vi "Main_25a.vi"() -> ()   [LabVIEW 2020]
uses:
  Cluster SNAFU Number.ctl
  ENUM_SNAFU Digit.ctl
  0fccf756-9261-4bff-9dad-ca374a7b94a1.vi
  <vilib>/Comparison/Equal/Equal Functor/Equal Functor.lvclass
panel:
  out "String":string
  in  "Example 2":string="1=-0-2\n12111\n2=0=\n21\n2=01\n111\n20012\n112\n1=-1=\n1-12\n12\n1=\n122"
  out "Array 2":T1[](array[typedef])
  out "Array":i64[](array[numeric])
  in  "Example":string="1=-0-2\n12111\n2=0=\n21\n2=01\n111\n20012\n112\n1=-1=\n1-12\n12\n1=\n122"
  in  "Decimal to SNAFU":string="Decimal          SNAFU\n        1              1\n        2              2\n        3             1=\n        4             1-\n        5             10\n        6             11\n        7             12\n        8             2=\n        9             2-\n       10             20\n       15            1=0\n       20            1-0\n     2022         1=11-2\n    12345        1-0---0\n314159265  1121-1110-1=0"
  out "Answer":i64
  in  "Puzzle":string="11-00\n2--2==212=12\n1=0110121=2\n1=012-21-=121\n1==0-1121-=200=2212\n1=1210===00=\n11210021-0001010-\n12=1-10-1-\n212-2==221-210-21\n1=-01=0-02-2-=-222=\n1=022000===-22010\n1=01=12202\n11=\n202-1\n2-12-2=--1\n10-=-00=101=-0-=-0\n1112-1\n2--1201\n1=1==-020=1-\n1--0-=2-0022-\n1=-1-21-200-102=\n11=100021210\n1=2=01=2-=01-=\n1=0120-11-0-=-2=-2\n1=-20221=2=-2=\n1-0\n1=00=-=11100--=2\n22122\n1=102222\n1210=1=001-=000\n1--200102022-=\n102=12=-1==\n100=\n20-02\n10\n10==-102\n11=020-0210-1-2012=\n12-11=0-1-=\n20=-\n212=1-1-10\n1=20=1-=2-11=0\n1=22\n120=2202=12200\n1-0-1\n211011-11=\n2=120=--==0==--0-0\n110-0-=-10-1-112\n1=2=1-=1-2\n1=12==10\n10=2110..."
  in  "SNAFU to Decimal":string="SNAFU  Decimal\n1=-0-2     1747\n 12111      906\n  2=0=      198\n    21       11\n  2=01      201\n   111       31\n 20012     1257\n   112       32\n 1=-1=      353\n  1-12      107\n    12        7\n    1=        3\n   122       37"
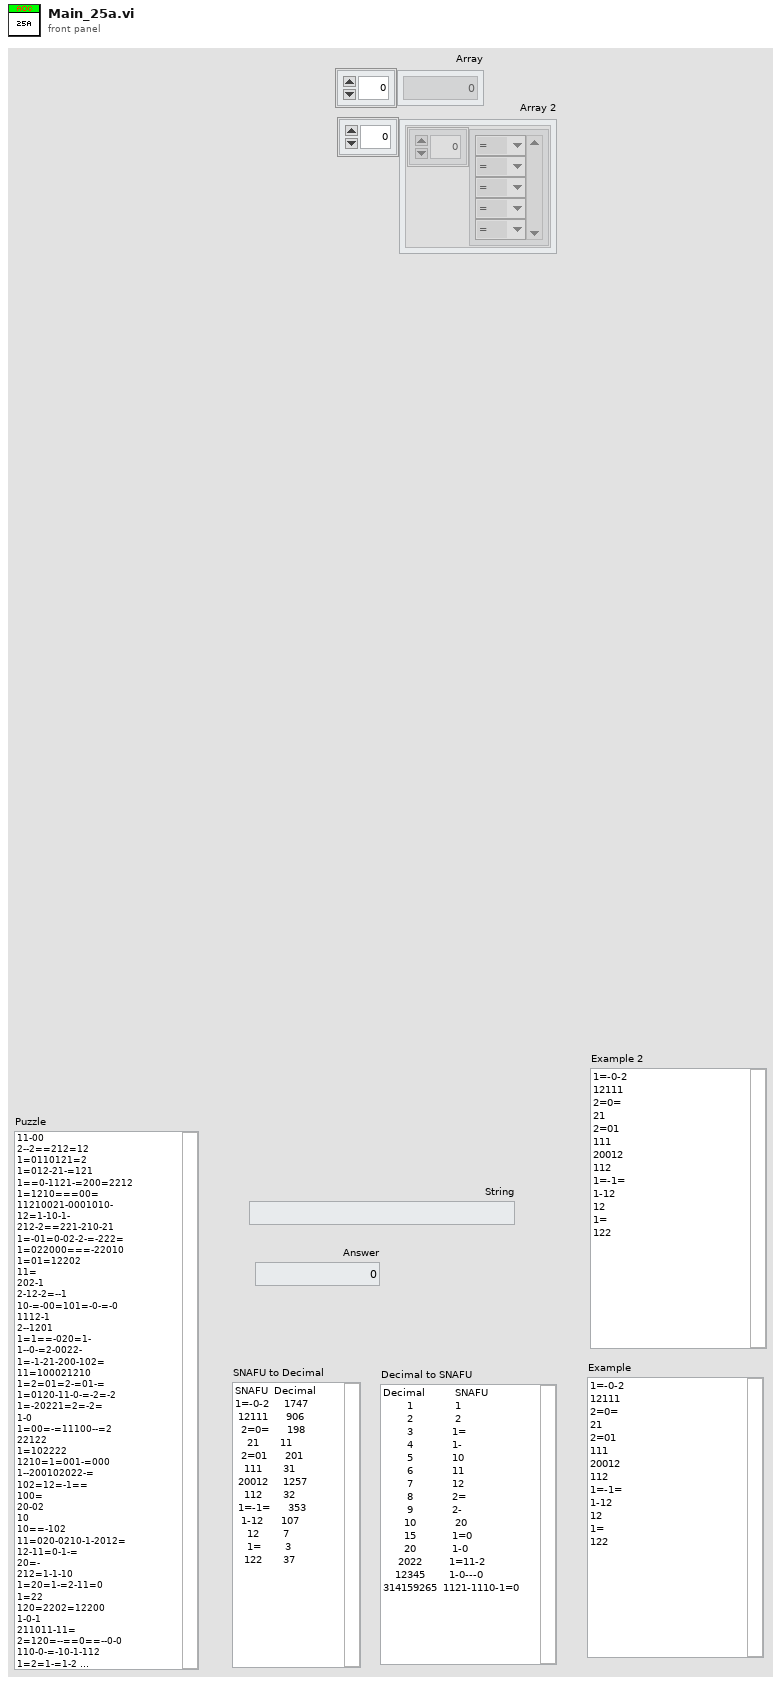
[diagram p1: front panel]
types:
  T1 = typedef "Cluster SNAFU Number.ctl" = cluster{"Digits":T2[]}
  T2 = typedef "ENUM_SNAFU Digit.ctl" = enum16{"=", "-", "0", "1", "2"}
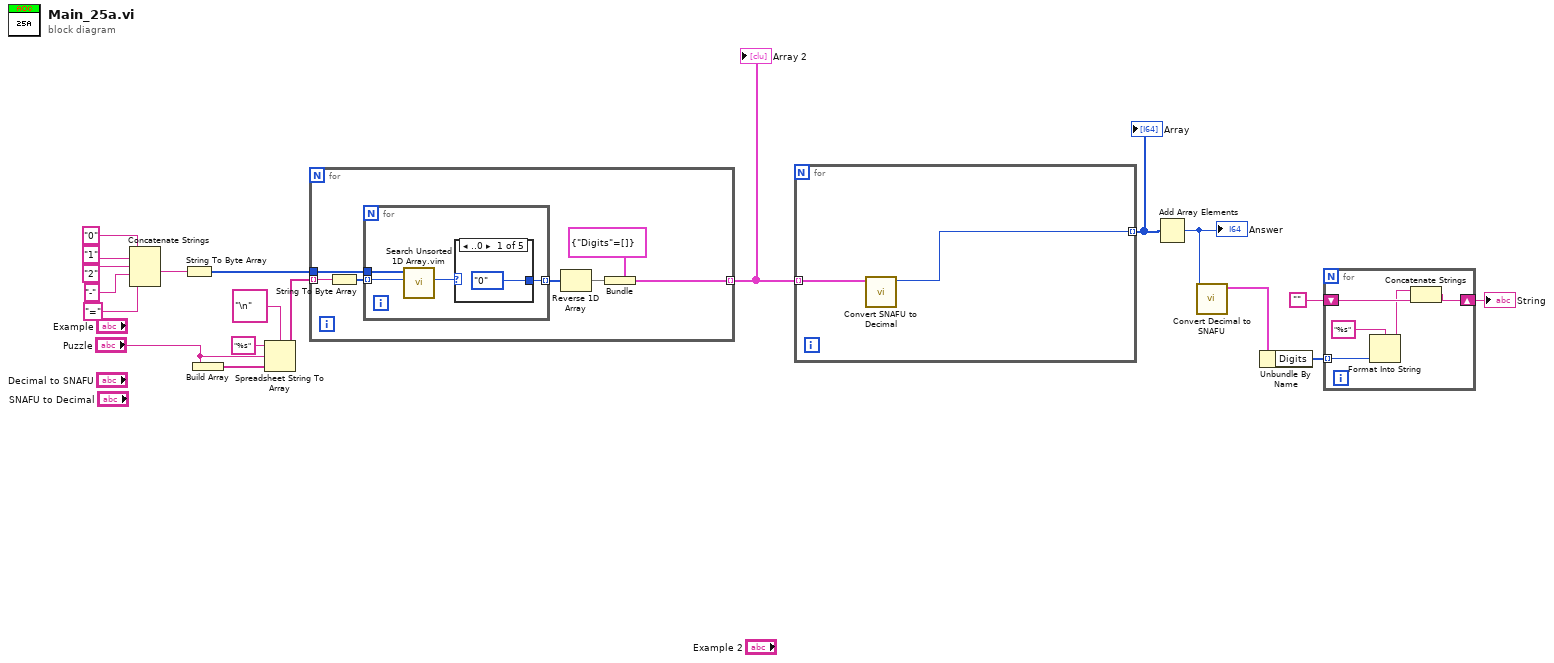
[diagram p0: block diagram]
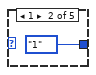
[diagram p2: hidden frame]
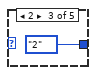
[diagram p3: hidden frame]
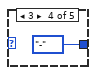
[diagram p4: hidden frame]
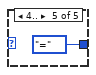
[diagram p5: hidden frame]
diagram:
  n1 = Concatenate Strings("0" ("Example"), "1" ("Example"), "2" ("Example"), "-" ("Example"), "=" ("Example")) -> (w10:string)
  n2 = String To Byte Array(string=w10) -> (unsigned byte array=w9:u8[])
  n3 = Build Array("Puzzle") -> (w19:string[])
  n4 = Spreadsheet String To Array(delimiter (Tab)="\n", format string="%s", spreadsheet string="Puzzle", array type (2D Dbl)=w19) -> (array=w16:string[])
  n5 = for {
    tunnel: w16 -> [w26] mode=indexing
    tunnel: w9 -> [w24]
    tunnel: [w21] -> w8 mode=indexing
    n6 = String To Byte Array(string=w26) -> (unsigned byte array=w25:u8[])
    n7 = for {
      tunnel: w25 -> [w29] mode=indexing
      tunnel: w24 -> [w30]
      tunnel: [w27] -> w23 mode=indexing
      n8 = call "Search Unsorted 1D Array.vim"("element"=w29, "unsorted 1D array"=w30) -> ("index of element"=w28:i32)  [unwired: 9 in]
      n9 = case shown="..0" w28 {
        tunnel: [ENUM_SNAFU_Digit."0" ("SNAFU IDs") ENUM_SNAFU_Digit."1" ("SNAFU IDs") ENUM_SNAFU_Digit."2" ("SNAFU IDs") ENUM_SNAFU_Digit."-" ("SNAFU IDs") ENUM_SNAFU_Digit."=" ("SNAFU IDs")] -> w27
        frame ..0 {
        }
        frame 1 {
        }
        frame 2 {
        }
        frame 3 {
        }
        frame 4.. {
        }
      }
    }
    n10 = Reverse 1D Array(array=w23) -> (reversed array=w22:T2[])
    n11 = Bundle(cluster=T1 {"Digits"=[]} ("Cluster"), "Digits"=w22) -> (w21:T1)
  }
  "Array 2" <- w8
  n12 = for {
    tunnel: w8 -> [w37] mode=indexing
    tunnel: [w36] -> w7 mode=indexing
    n13 = call "Convert SNAFU to Decimal.vi"("Cluster"=w37) -> ("Decimal"=w36:i64)  [unwired: 10 in]
  }
  "Array" <- w7
  n14 = Add Array Elements(numeric array=w7) -> (sum=w6:i64)
  "Answer" <- w6
  n15 = call "Convert Decimal to SNAFU.vi"("Decimal"=w6) -> ("SNAFU Number"=w5:T1)  [unwired: 10 in]
  n16 = Unbundle By Name(w5) -> ("Digits"=w4:T2[])
  n17 = for {
    tunnel: w4 -> [w42] mode=indexing
    shift-right: [w39] -> w2
    shift-left: "" -> [w40]
    n18 = Format Into String(format string="%s", w42) -> (resulting string=w38:string)  [unwired: 2 in, 1 out]
    n19 = Concatenate Strings(w38, w40) -> (w39:string)
  }
  "String" <- w2
